vi "FlatToRichnixnet_grpc_GetSubPropertyResponse.vi"(5 "OutputClusterType":T1, 11 "InputCluster":T2) -> (3 "OutputCluster":T1)   [LabVIEW 2025, in "grpc-xnet_client.lvlib"]
uses:
  grpc-xnet_client.lvlib
  nixnet_grpc_GetSubPropertyResponse_Flat.ctl
  nixnet_grpc_GetSubPropertyResponse.ctl
  nixnet_grpc_GetSubPropertyResponse_property_value/nixnet_grpc_GetSubPropertyResponse_property_value.lvclass
  nixnet_grpc_GetSubPropertyResponse_property_value/nixnet_grpc_GetSubPropertyResponse_property_value.lvclass/nixnet_grpc_GetSubPropertyResponse_property_value.ctl
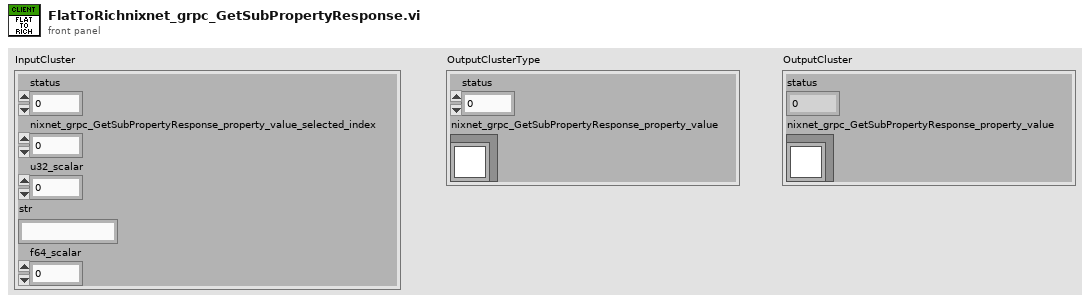
[diagram p1: front panel]
types:
  T1 = typedef "grpc-xnet_client.lvlib/nixnet_grpc_GetSubPropertyResponse.ctl" = cluster{"status":i32, "nixnet_grpc_GetSubPropertyResponse_property_value":refnum<class "nixnet_grpc_GetSubPropertyResponse_property_value.lvclass">}
  T2 = typedef "grpc-xnet_client.lvlib/nixnet_grpc_GetSubPropertyResponse_Flat.ctl" = cluster{"status":i32, "nixnet_grpc_GetSubPropertyResponse_property_value_selected_index":i32, "u32_scalar":u32, "str":string, "f64_scalar":dbl}
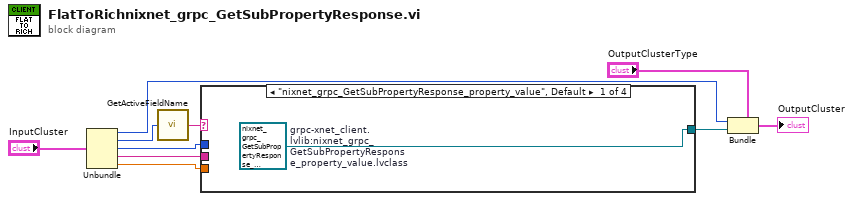
[diagram p0: block diagram]
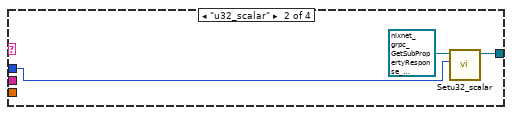
[diagram p2: hidden frame]
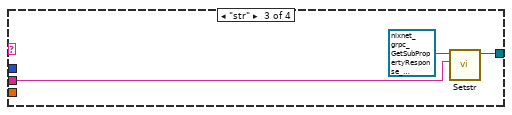
[diagram p3: hidden frame]
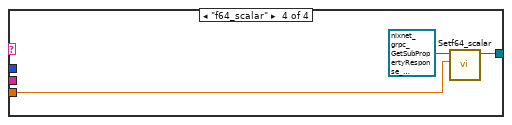
[diagram p4: hidden frame]
diagram:
  n1 = Unbundle "Unbundle"("InputCluster") -> ("status"=w7:i32, "nixnet_grpc_GetSubPropertyResponse_property_value_selected_index"=w6:i32, "u32_scalar"=w3:u32, "str"=w2:string, "f64_scalar"=w1:dbl)
  n2 = call "GetActiveFieldName.vi"("protobuf index"=w6) -> ("oneof field name"=w5:string)
  n3 = case "nixnet_grpc_GetSubPropertyResponse_property_value" shown="\"nixnet_grpc_GetSubPropertyResponse_property_value\", Default" w5 {
    tunnel: [w11 w13 w16 w19] -> w4
    tunnel: w3 -> [_ w14 _ _]
    tunnel: w2 -> [_ _ w17 _]
    tunnel: w1 -> [_ _ _ w20]
    frame "nixnet_grpc_GetSubPropertyResponse_property_value", Default {
      w11 = refnum<class "nixnet_grpc_GetSubPropertyResponse_property_value.lvclass"> refnum  # grpc-xnet_client.lvlib:nixnet_grpc_GetSubPropertyResponse_property_value.lvclass
    }
    frame "u32_scalar" {
      n4 = call "Setu32_scalar.vi"("Set_Val"=w14, "OneOfTemplate in"=refnum<class "nixnet_grpc_GetSubPropertyResponse_property_value.lvclass"> refnum) -> ("OneOfTemplate out"=w13:refnum<class "nixnet_grpc_GetSubPropertyResponse_property_value.lvclass">)  [unwired: 8 in, 1 out]
    }
    frame "str" {
      n5 = call "Setstr.vi"("Set_Val"=w17, "OneOfTemplate in"=refnum<class "nixnet_grpc_GetSubPropertyResponse_property_value.lvclass"> refnum) -> ("OneOfTemplate out"=w16:refnum<class "nixnet_grpc_GetSubPropertyResponse_property_value.lvclass">)  [unwired: 8 in, 1 out]
    }
    frame "f64_scalar" {
      n6 = call "Setf64_scalar.vi"("Set_Val"=w20, "OneOfTemplate in"=refnum<class "nixnet_grpc_GetSubPropertyResponse_property_value.lvclass"> refnum) -> ("OneOfTemplate out"=w19:refnum<class "nixnet_grpc_GetSubPropertyResponse_property_value.lvclass">)  [unwired: 8 in, 1 out]
    }
  }
  n7 = Bundle "Bundle"(cluster="OutputClusterType", "status"=w7, "nixnet_grpc_GetSubPropertyResponse_property_value"=w4) -> (→"OutputCluster":T1)
